vi "Write Value.vi"(8 "error in (no error)":errorcluster, 10 "Data":T1, 11 "Numeric in":refnum<class "Const_EXT.lvclass">) -> (0 "error out":errorcluster, 3 "Numeric out":refnum<class "Const_EXT.lvclass">)   [LabVIEW 2021, in "Const_EXT.lvclass"]
uses:
  Const_EXT.lvclass
  Type.ctl
  Const_EXT.lvclass/Const_EXT.ctl
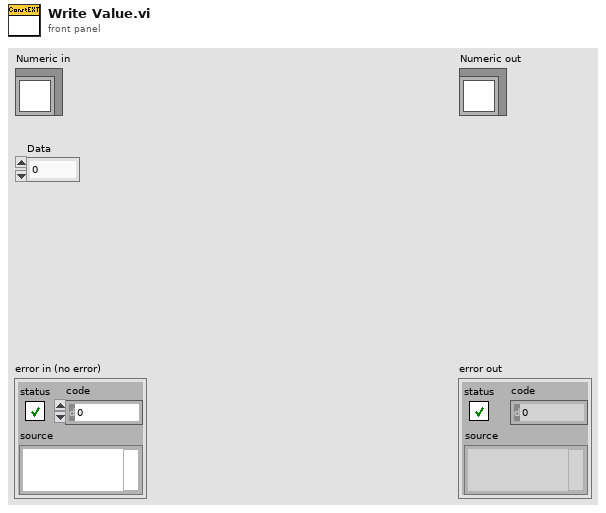
[diagram p1: front panel]
types:
  T1 = typedef "Const_EXT.lvclass/Type.ctl" = ext
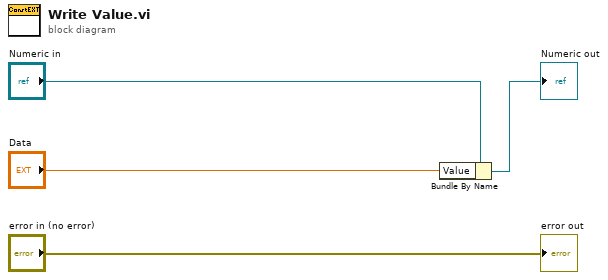
[diagram p0: block diagram]
diagram:
  n1 = Bundle By Name(cluster="Numeric in", "Value"="Data") -> (→"Numeric out":refnum<class "Const_EXT.lvclass">)
  "error out" <- "error in (no error)"
